vi "daq_sonar_output.vi"() -> ()   [LabVIEW 2011]
panel:
  in  "physical channels":tag
  out "Output (inches)":dbl
  out "error out":errorcluster
  in  "VCC (default 5)":dbl=5.0
  in  "stop":bool
  in  "error in":errorcluster
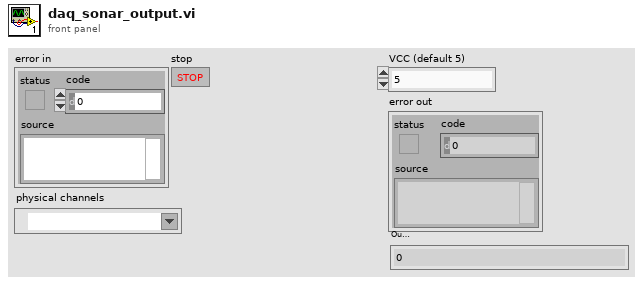
[diagram p1: front panel]
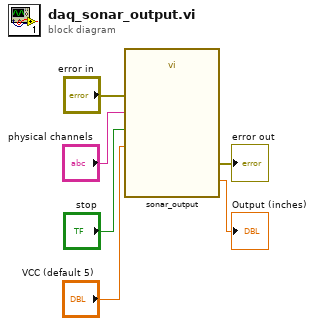
[diagram p0: block diagram]
diagram:
  n1 = call "sonar_output.vi"("stop"="stop", "error in"="error in", "VCC (default 5)"="VCC (default 5)", "physical channels"="physical channels") -> ("error out"=→"error out":errorcluster, "Output (inches)"=→"Output (inches)":dbl)  [unwired: 6 in]
